vi "Direction agnostic read volume and status.vi"(0 "VISA resource name":refnum<visa-resource-name>="COM1", 5 "Address (00)":i32 format="%02.0f", 11 "error in (no error)":errorcluster) -> (3 "Vol OK?":bool, 4 "VISA resource name out":refnum<visa-resource-name>, 6 "Volume":dbl, 8 "Units":string, 10 "Pump status":T1 items=["Error - Can't read status"=-1, "Stopped"=0, "Infusing"=1, "Withdrawing"=2, "Pump stalled"=3, "Stopped at infuse limit"=4, "Stopped at withdraw limit"=5, "Emergency stop"=6, "Stopped at target volume"=7], 13 "Total volume withdrawn since clear":dbl, 14 "Total volume infused since clear":dbl, 15 "error out":errorcluster)   [LabVIEW 2015]
doc: "This VI returns the current acuumulated *net* withdrawn volume, units in ml or ul depending on range, and the pump status.\n\nModified from original which is Copyright 2005, National Instruments Corporation.\n\nModifications Copyright 2009, Jeff Gelles, Brandeis University"
uses:
  Pump status.ctl
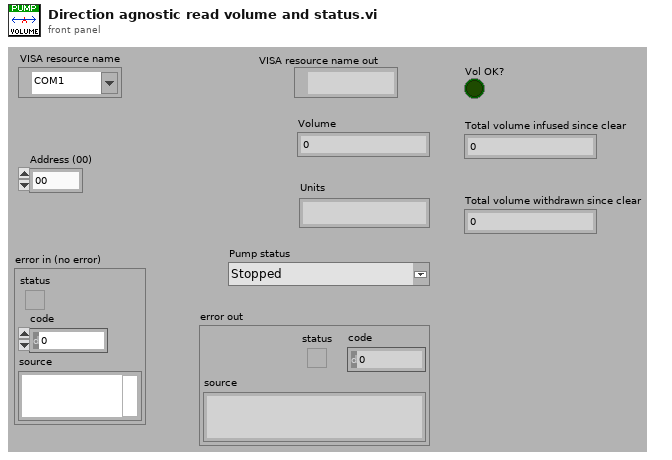
[diagram p1: front panel]
types:
  T1 = typedef "Pump status.ctl" = i8
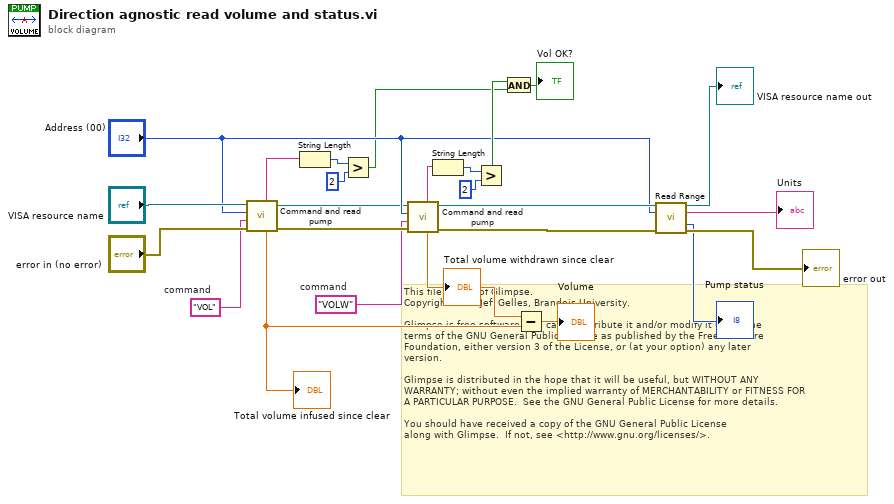
[diagram p0: block diagram]
diagram:
  w9 = "VOL"  # command
  w8 = "VOLW"  # command
  # "This file is part of Glimpse. \nCopyright 2014 Jeff Gelles, Brandeis University.    \n\nGlimpse is free software: you can redistribute it and/or modify it under the \nterms of the GNU General Public License as published by the Free Software \nFoundation, either version 3 of the License, or (at your option) any later \nversion.\n\nGlimpse is distributed in the hope that it will be useful, but WITHOUT ANY \nWARRANTY; without even the implied warranty of MERCHANTABILITY or FITNESS FOR \nA PARTICULAR PURPOSE.  See the GNU General Public License for more details.\n\nYou should have received a copy of the GNU General Public License\nalong with Glimpse.  If not, see <http://www.gnu.org/licenses/>."
  n1 = call "Command and read pump.vi"("error in (no error)"="error in (no error)", "command"=w9, "Address (00)"="Address (00)", "VISA resource name"="VISA resource name") -> ("error out"=w12:errorcluster, "VISA resource name out"=w11:refnum<visa-resource-name>, "Numeric result"=w1:dbl, "String result"=w5:string)  [unwired: 4 out]
  "Total volume infused since clear" <- w1
  n2 = String Length(string=w5) -> (length=w6:i32)
  n3 = Greater?(x=w6, y=2) -> (0:w3:bool)
  n4 = call "Command and read pump.vi"("error in (no error)"=w12, "command"=w8, "Address (00)"="Address (00)", "VISA resource name"=w11) -> ("error out"=w24:errorcluster, "VISA resource name out"=w25:refnum<visa-resource-name>, "Numeric result"=w2:dbl, "String result"=w19:string)  [unwired: 4 out]
  "Total volume withdrawn since clear" <- w2
  n5 = String Length(string=w19) -> (length=w18:i32)
  n6 = Greater?(x=w18, y=2) -> (0:w16:bool)
  n7 = And(x=w16, y=w3) -> (x .and. y?=→"Vol OK?":bool)
  n8 = Subtract(x=w2, y=w1) -> (x-y=→"Volume":dbl)
  n9 = call "Read Range.vi"("VISA resource name"=w25, "Address (00)"="Address (00)", "error in (no error)"=w24) -> ("VISA resource name out"=→"VISA resource name out":refnum<visa-resource-name>, "Target Units"=→"Units":string, "Pump status"=→"Pump status":T1, "error out"=→"error out":errorcluster)  [unwired: 9 out]
